vi "DecodeJPEGString.vi"(4 "error in":errorcluster, 6 "Compressed Image":string, 7 "Image In":T1) -> (0 "error out":errorcluster, 3 "Image Out":T1)   [LabVIEW 2017]
uses:
  <vilib>/vision/Image Controls.llb/IMAQ Image.ctl
  nivissvc.dll
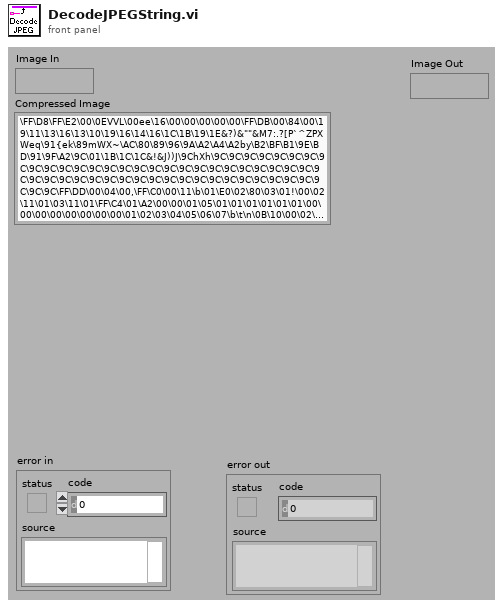
[diagram p1: front panel]
types:
  T1 = typedef "IMAQ Image.ctl" = refnum<image>
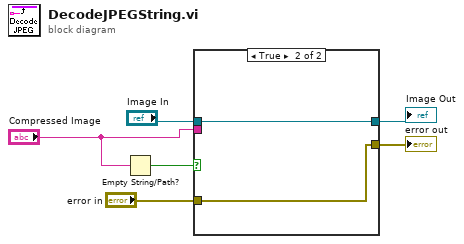
[diagram p0: block diagram]
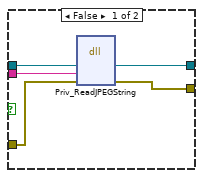
[diagram p2: hidden frame]
diagram:
  n1 = Empty String/Path?(string/path="Compressed Image") -> (empty?=w1:bool)
  n2 = case shown="True" w1 {
    tunnel: "Compressed Image" -> [w11 _]
    tunnel: "Image In" -> [w10 w13]
    tunnel: "error in" -> [w9 w12]
    tunnel: [w8 w12] -> w4
    tunnel: [w7 w13] -> w3
    frame False {
      n3 = dll-call lib="nivissvc.*" fn="Priv_ReadJPEGString"("image"=w10, "name"=w11, "err"=w9) -> ("image"=w7:T1, "err"=w8:errorcluster)  [unwired: 5 in, 2 out]
    }
    frame True {
    }
  }
  "error out" <- w4
  "Image Out" <- w3
